vi "alligning data.vi"() -> (1 "Second part":waveform(dbl)[](graph), 2 "First Part":waveform(dbl)[](graph))   [LabVIEW 2020]
uses:
  <vilib>/measure/maresamp.llb/Resample Waveform (single shot).vi
  <vilib>/measure/maspectr.llb/FFT Spectrum (Real-Im) for 1 Chan.vi
  <vilib>/measure/NI_MAPro.lvlib
panel:
  out "Waveform Graph 6":cluster{"f0":dbl, "df":dbl, "real part":dbl[]}(graph)
  out "Delta second part 2":dbl
  out "Delta first part 2":dbl
  out "Delta second part":dbl
  out "Delta first part":dbl
  in  "Tab Control":enum32{"Page 1", "Page 3", "Page 4", "Page 2"}(tab)
  out "Waveform Graph 2":waveform(dbl)[](graph)
  out "Waveform Graph 3":waveform(dbl)[](graph)
  out "Array 4":i32[](array[numeric])
  out "Array 5":i32[](array[numeric])
  out "Waveform Graph 5":waveform(dbl)[](graph)
  out "Waveform Graph 4":waveform(dbl)[](graph)
  out "Array 2":i32[](array[numeric])
  out "Array 3":i32[](array[numeric])
  out "Array 7":i32[](array[numeric])
  out "Array 6":i32[](array[numeric])
  out "lv split cut":i32
  out "ex split cut":i32
  out "First ex cut":i32
  out "second subarray 2":dbl[](array[numeric])
  out "first subarray 2":dbl[](array[numeric])
  out "second subarray":dbl[](array[numeric])
  out "first subarray":dbl[](array[numeric])
  out "Array":i32[](array[numeric])
  out "x-y":dbl
  # "LV\nEX\nNew"
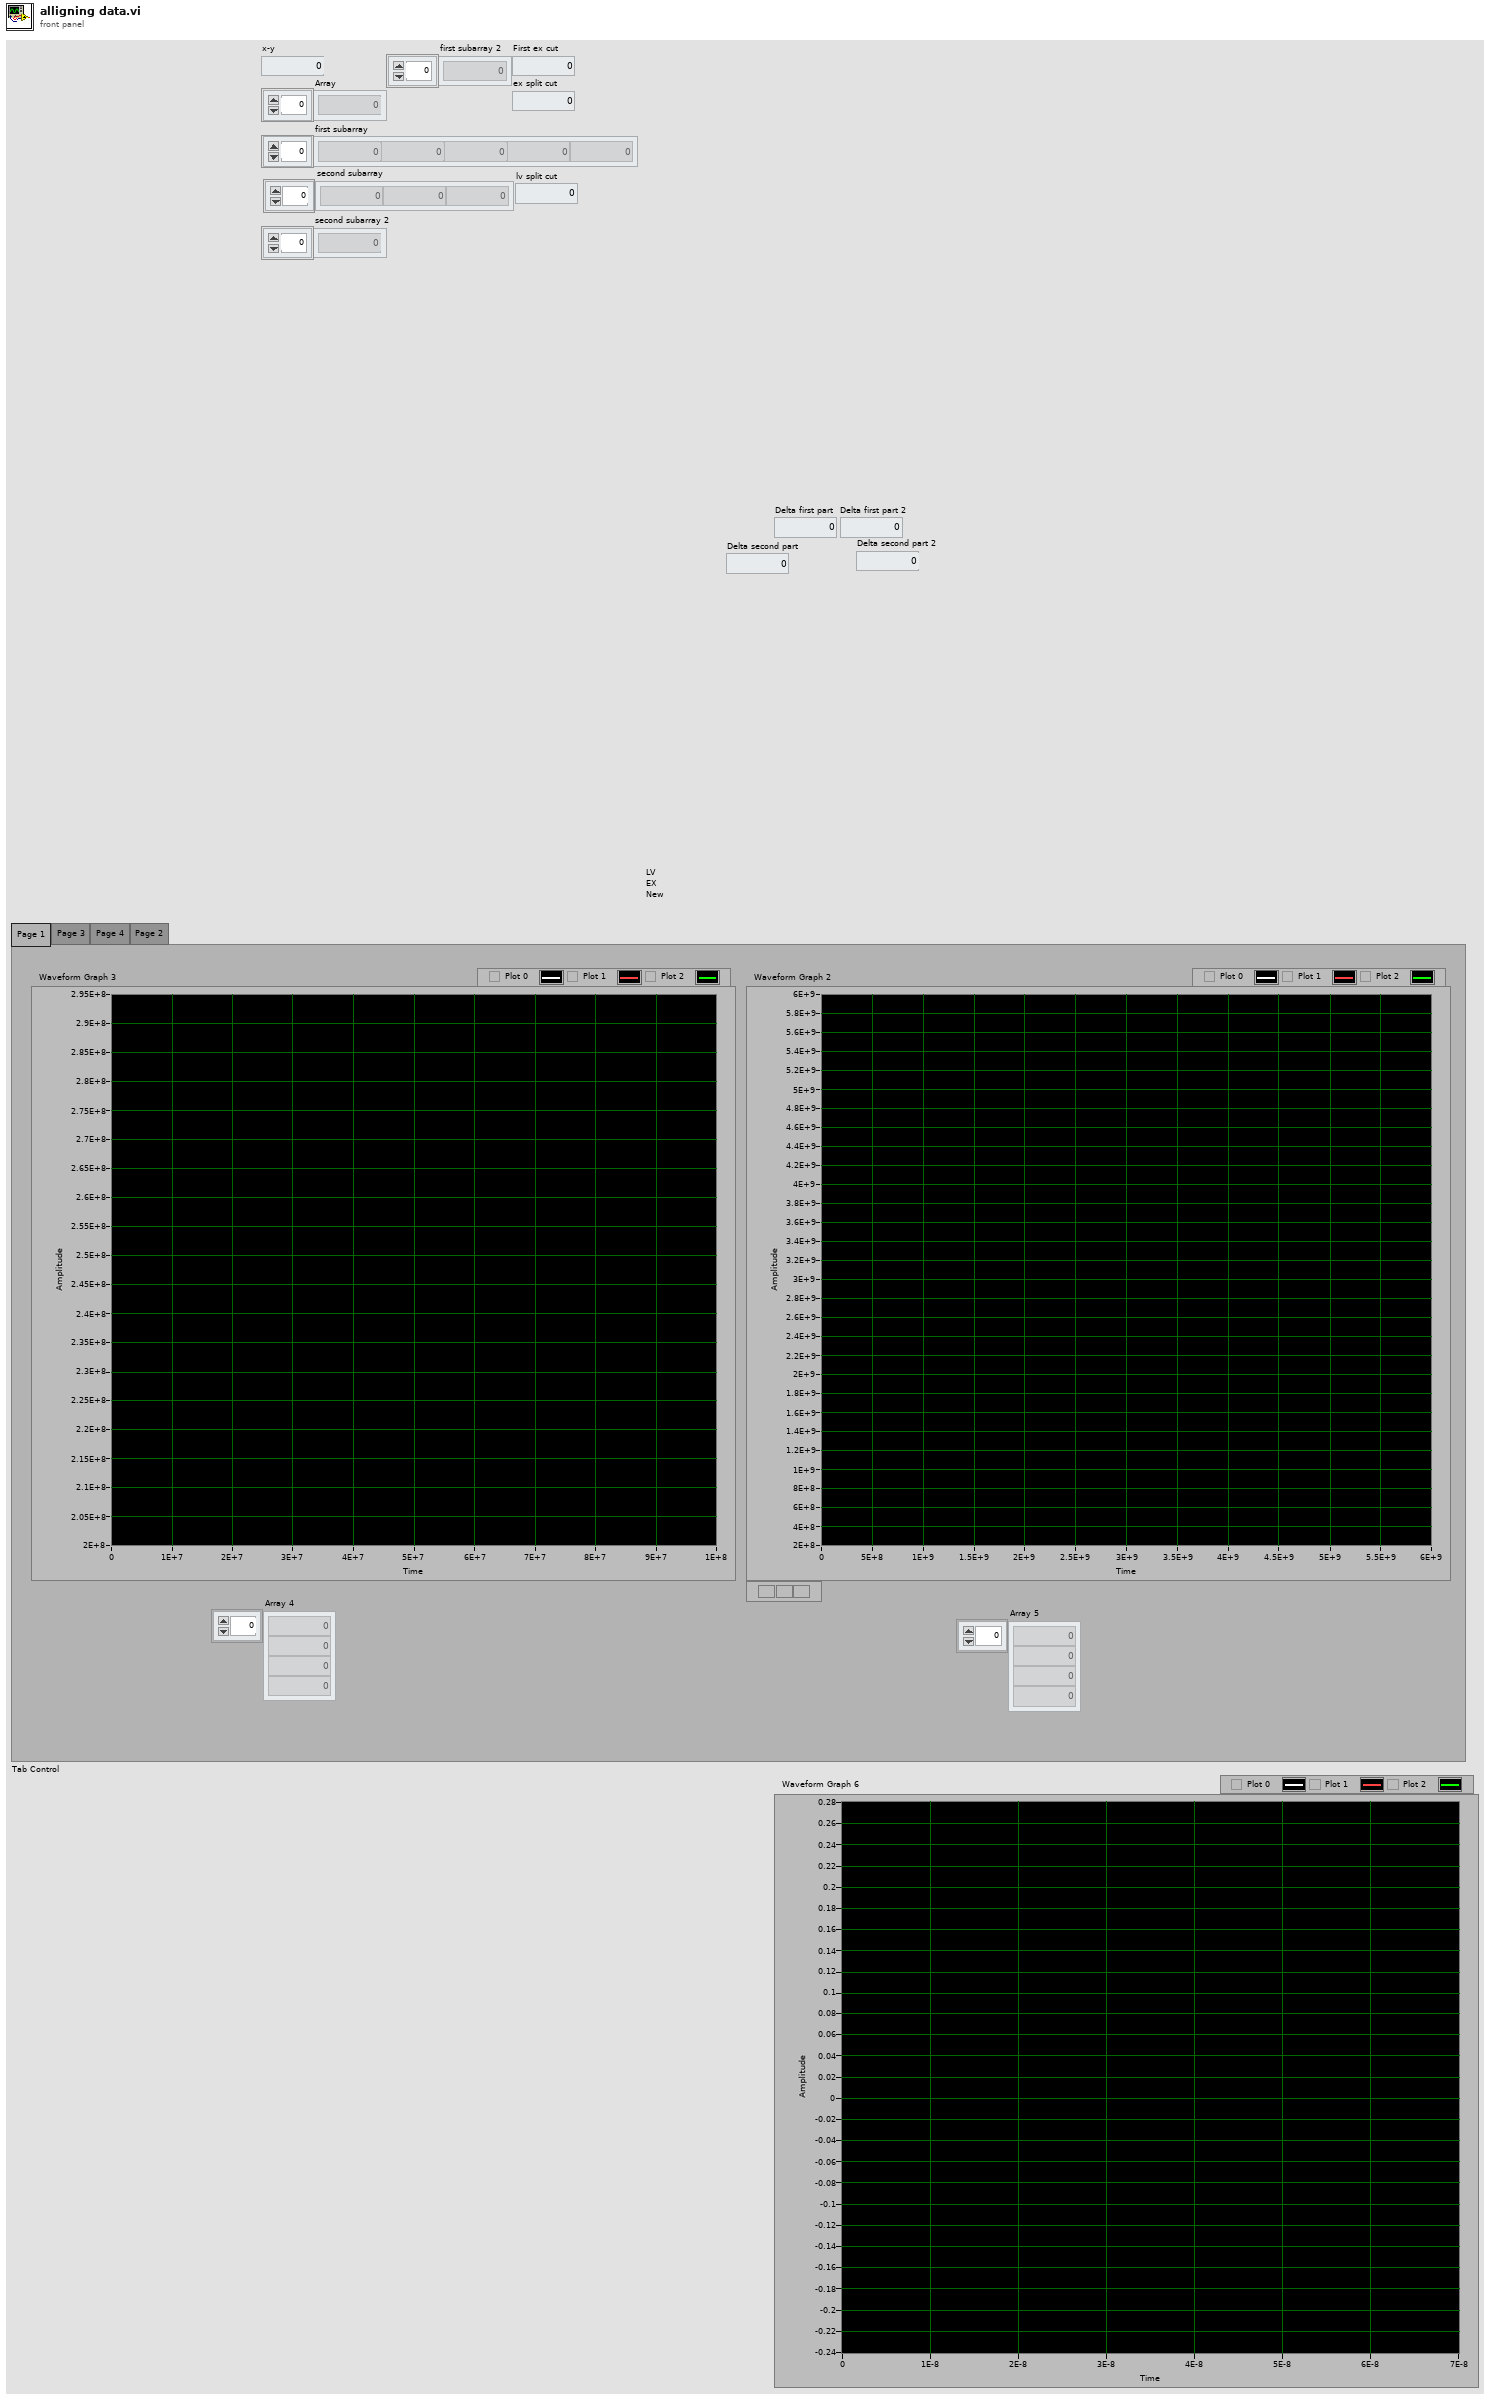
[diagram p1: front panel]
types:
  T1 = typedef "VFH-VNA_File_Handler.lvlib/VFH-file_cluster-Expensive.ctl" = cluster{"Frequency":dbl[], "Permativity'":dbl[], "Permativity''":dbl[], "Q [S/m]":dbl[], "Tan":dbl[], "Reflection R":dbl[], "Reflection I":dbl[]}
  T2 = typedef "VFH-VNA_File_Handler.lvlib/VFH-file_cluster-NanoVNA.ctl" = cluster{"Frequency":dbl[], "S11_Real":dbl[], "S11_Imag":dbl[], "S21_Real":dbl[], "S21_Imag":dbl[], "S12_Real":dbl[], "S12_Imag":dbl[], "S22_Real":dbl[], "S22_Imag":dbl[]}
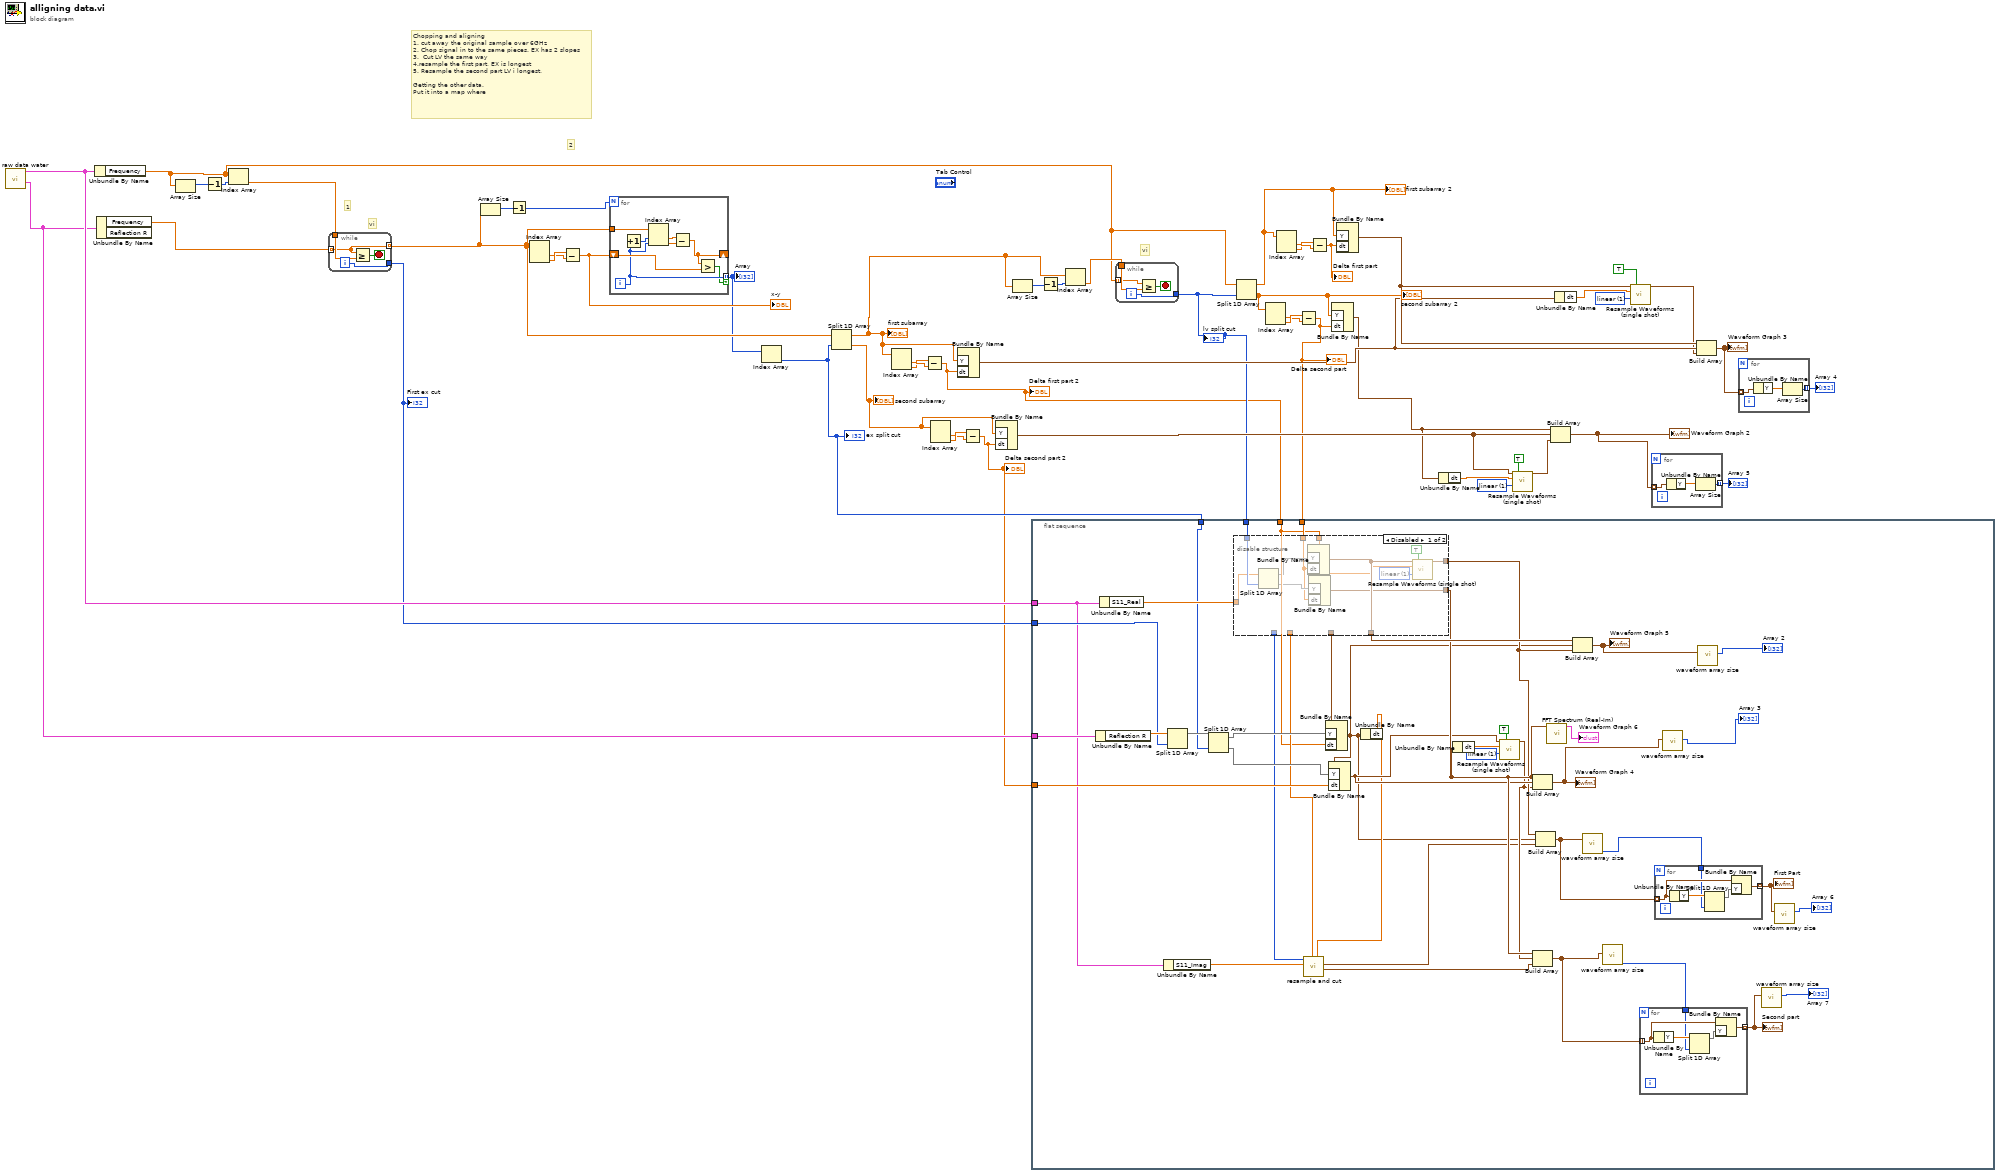
[diagram p0: block diagram]
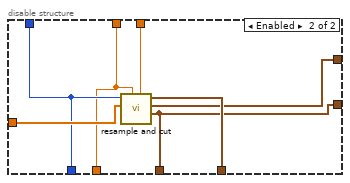
[diagram p2: hidden frame]
diagram:
  w17 = u16 1 items=["coerce", "linear", "spline", "FIR filter"] ("interpolation mode")
  w23 = u16 1 items=["coerce", "linear", "spline", "FIR filter"] ("interpolation mode")
  # "vi"
  # "vi"
  # "2"
  # "1"
  # "Chopping and aligning\n1. cut away the original sample over 6GHz \n2. Chop signal in to the same pieces. EX has 2 slopes\n3.  Cut LV the same way\n4.resample the first part, EX is longest\n5. Resample the second part LV i longest.\n\nGetting the other data.\nPut it into a map where"
  n1 = call "raw data water.vi"() -> ("output R140"=w11:T1, "avg output NV"=w12:T2)  [unwired: 9 in, 1 out]
  n2 = Unbundle By Name(w12) -> ("Frequency"=w38:dbl[])
  n3 = Unbundle By Name(w11) -> ("Frequency"=w49:dbl[])  [unwired: 1 out]
  n4 = Array Size(array=w38) -> (size(s)=w52:i32)
  n5 = Decrement(x=w52) -> (x-1=w51:i32)
  n6 = Index Array(array=w38, index=w51) -> (element=w50:dbl)
  n7 = while {
    tunnel: w49 -> [w54] mode=indexing
    tunnel: w50 -> [w56]
    tunnel: [w54] -> w43 mode=indexing
    tunnel: [w53] -> w10
    i -> [w53]
    stop <- w55 stop-if-true
    n8 = Greater Or Equal?(x=w54, y=w56) -> (x >= y?=w55:bool)
  }
  "First ex cut" <- w10
  n9 = Array Size(array=w43) -> (size(s)=w45:i32)
  n10 = Decrement(x=w45) -> (x-1=w44:i32)
  n11 = Index Array(array=w43) -> (element #1=w47:dbl, element #2=w48:dbl)  [unwired: 2 in]
  n12 = Subtract(x=w48, y=w47) -> (x-y=w46:dbl)
  "x-y" <- w46
  n13 = for {
    N: w44 -> [_]
    tunnel: w43 -> [w64]
    shift-right: [w60] -> _
    shift-left: w46 -> [w59]
    tunnel: [w58] -> w42 mode=indexing if=w57
    i -> [w58]
    n14 = Increment(x=w58) -> (x+1=w63:i32)
    n15 = Index Array(array=w64, index #1=w63, index #2=w58) -> (element #1=w62:dbl, element #2=w61:dbl)
    n16 = Subtract(x=w62, y=w61) -> (x-y=w60:dbl)
    n17 = Greater?(x=w60, y=w59) -> (0:w57:bool)
  }
  "Array" <- w42
  n18 = Index Array(array=w42) -> (element=w9:i32)  [unwired: 1 in]
  "ex split cut" <- w9
  n19 = Split 1D Array(array=w43, index=w9) -> (first subarray=w28:dbl[], second subarray=w25:dbl[])
  "first subarray" <- w28
  "second subarray" <- w25
  n20 = Index Array(array=w28) -> (element #1=w30:dbl, element #2=w29:dbl)  [unwired: 2 in]
  n21 = Subtract(x=w29, y=w30) -> (x-y=w6:dbl)
  "Delta first part 2" <- w6
  n22 = Index Array(array=w25) -> (element #1=w26:dbl, element #2=w27:dbl)  [unwired: 2 in]
  n23 = Bundle By Name("Y"=w28, "dt"=w6) -> (w21:waveform(dbl))  [unwired: 1 in]
  n24 = Subtract(x=w27, y=w26) -> (x-y=w5:dbl)
  "Delta second part 2" <- w5
  n25 = Bundle By Name("Y"=w25, "dt"=w5) -> (w15:waveform(dbl))  [unwired: 1 in]
  n26 = Array Size(array=w28) -> (size(s)=w40:i32)
  n27 = flat-sequence {
    tunnel: w12 -> [w75]
    tunnel: w11 -> [w106]
    tunnel: w10 -> [w94]
    tunnel: w9 -> [w93]
    tunnel: w8 -> [w98]
    tunnel: w7 -> [w103]
    tunnel: w6 -> [w68]
    tunnel: w5 -> [w102]
    frame #0 {
      w100 = u16 1 items=["coerce", "linear", "spline", "FIR filter"] ("interpolation mode")
      n28 = Unbundle By Name(w106) -> ("Reflection R"=w95:dbl[])
      n29 = Unbundle By Name(w75) -> ("S11_Real"=w97:dbl[])
      n30 = Unbundle By Name(w75) -> ("S11_Imag"=w74:dbl[])
      n31 = Split 1D Array(array=w95, index=w94) -> (first subarray=w96:dbl[])  [unwired: 1 out]
      n32 = Split 1D Array(array=w96, index=w93) -> (first subarray=w104:dbl[], second subarray=w105:dbl[])
      n33 = disable-structure shown="Disabled" {
        disable-tunnel: w103 -> [w113 w120]
        disable-tunnel: w98 -> [w112 w121]
        disable-tunnel: w97 -> [w111 w124]
        disable-tunnel: [w110 w123] -> w91
        disable-tunnel: [w109 w118] -> w90
        disable-tunnel: [w108 w122] -> w88
        disable-tunnel: [_ w121] -> w73
        disable-tunnel: [_ w120] -> w72
        disable-tunnel: w68 -> [w107 w119]
        disable-tunnel: [_ w118] -> w67
        frame Disabled {
          w114 = u16 1 items=["coerce", "linear", "spline", "FIR filter"] ("interpolation mode")
          n34 = Split 1D Array(array=w111, index=w112) -> (first subarray=w117:dbl[], second subarray=w116:dbl[])
          n35 = Bundle By Name("Y"=w117, "dt"=w113) -> (w110:waveform(dbl))  [unwired: 1 in]
          n36 = Bundle By Name("Y"=w116, "dt"=w113) -> (w109:waveform(dbl))  [unwired: 1 in]
          n37 = call-poly <vilib>:"Resample Waveforms (single shot).vi"("waveform in"=w110, "open interval? (F)"=TRUE, "dt"=w107, "interpolation mode"=w114) -> ("resampled waveform out"=w108:waveform(dbl))  [unwired: 8 in, 3 out]
        }
        frame Enabled {
          n38 = call "resample and cut.vi"("new dt"=w119, "signal dt"=w120, "array"=w124, "Splite"=w121) -> ("org second part"=w118:waveform(dbl), "resampled first part"=w122:waveform(dbl), "Org first part"=w123:waveform(dbl))  [unwired: 5 in]
        }
      }
      n39 = Bundle By Name(cluster=w67, "Y"=w104, "dt"=w68) -> (w66:waveform(dbl))
      n40 = Bundle By Name(cluster=w66, "Y"=w105, "dt"=w102) -> (w89:waveform(dbl))
      n41 = Unbundle By Name(w66) -> ("dt"=w71:dbl)
      n42 = call "resample and cut.vi"("new dt"=w71, "signal dt"=w72, "array"=w74, "Splite"=w73) -> ("org second part"=w69:waveform(dbl), "resampled first part"=w70:waveform(dbl))  [unwired: 5 in, 1 out]
      n43 = Unbundle By Name(w90) -> ("dt"=w101:dbl)
      n44 = call-poly <vilib>:"Resample Waveforms (single shot).vi"("waveform in"=w89, "open interval? (F)"=TRUE, "dt"=w101, "interpolation mode"=w100) -> ("resampled waveform out"=w87:waveform(dbl))  [unwired: 8 in, 3 out]
      n45 = Build Array(w90, w87, w69) -> (w81:waveform(dbl)[])
      n46 = Build Array(w90, w89, w87) -> (w84:waveform(dbl)[])
      "Waveform Graph 4" <- w84
      n47 = Build Array(w88, w66, w70) -> (w82:waveform(dbl)[])
      n48 = call-poly <vilib>:"FFT Spectrum (Real-Im).vi"("time signal"=w90) -> ("real part"=→"Waveform Graph 6":cluster{"f0":dbl, "df":dbl, "real part":dbl[]})  [unwired: 6 in, 4 out]
      n49 = Build Array(w91, w66, w88) -> (w86:waveform(dbl)[])
      "Waveform Graph 5" <- w86
      n50 = call "waveform array size.vi"("Waveform"=w82) -> ("min value"=w65:i32)  [unwired: 8 in, 2 out]
      n51 = call "waveform array size.vi"("Waveform"=w81) -> ("min value"=w80:i32)  [unwired: 8 in, 2 out]
      n52 = for {
        tunnel: w81 -> [w129] mode=indexing
        tunnel: w80 -> [w126]
        tunnel: [w125] -> w77 mode=indexing
        n53 = Unbundle By Name(w129) -> ("Y"=w128:dbl[])
        n54 = Split 1D Array(array=w128, index=w126) -> (first subarray=w127:dbl[])  [unwired: 1 out]
        n55 = Bundle By Name(cluster=w129, "Y"=w127) -> (w125:waveform(dbl))
      }
      "Second part" <- w77
      n56 = for {
        tunnel: w82 -> [w134] mode=indexing
        tunnel: w65 -> [w131]
        tunnel: [w130] -> w79 mode=indexing
        n57 = Unbundle By Name(w134) -> ("Y"=w133:dbl[])
        n58 = Split 1D Array(array=w133, index=w131) -> (first subarray=w132:dbl[])  [unwired: 1 out]
        n59 = Bundle By Name(cluster=w134, "Y"=w132) -> (w130:waveform(dbl))
      }
      "First Part" <- w79
      n60 = call "waveform array size.vi"("Waveform"=w84) -> ("Array"=→"Array 3":i32[])  [unwired: 8 in, 2 out]
      n61 = call "waveform array size.vi"("Waveform"=w86) -> ("Array"=→"Array 2":i32[])  [unwired: 8 in, 2 out]
      n62 = call "waveform array size.vi"("Waveform"=w77) -> ("Array"=→"Array 7":i32[])  [unwired: 8 in, 2 out]
      n63 = call "waveform array size.vi"("Waveform"=w79) -> ("Array"=→"Array 6":i32[])  [unwired: 8 in, 2 out]
    }
  }
  n64 = Decrement(x=w40) -> (x-1=w41:i32)
  n65 = Index Array(array=w28, index=w41) -> (element=w39:dbl)
  n66 = while {
    tunnel: w38 -> [w136] mode=indexing
    tunnel: w39 -> [w138]
    tunnel: [w135] -> w8
    i -> [w135]
    stop <- w137 stop-if-true
    n67 = Greater Or Equal?(x=w136, y=w138) -> (x >= y?=w137:bool)
  }
  "lv split cut" <- w8
  n68 = Split 1D Array(array=w38, index=w8) -> (first subarray=w33:dbl[], second subarray=w31:dbl[])
  "first subarray 2" <- w33
  "second subarray 2" <- w31
  n69 = Index Array(array=w31) -> (element #1=w34:dbl, element #2=w35:dbl)  [unwired: 2 in]
  n70 = Index Array(array=w33) -> (element #1=w37:dbl, element #2=w36:dbl)  [unwired: 2 in]
  n71 = Subtract(x=w35, y=w34) -> (x-y=w7:dbl)
  "Delta second part" <- w7
  n72 = Subtract(x=w36, y=w37) -> (x-y=w32:dbl)
  "Delta first part" <- w32
  n73 = Bundle By Name("Y"=w31, "dt"=w7) -> (w14:waveform(dbl))  [unwired: 1 in]
  n74 = Bundle By Name("Y"=w33, "dt"=w32) -> (w22:waveform(dbl))  [unwired: 1 in]
  n75 = Unbundle By Name(w14) -> ("dt"=w18:dbl)
  n76 = call-poly <vilib>:"Resample Waveforms (single shot).vi"("waveform in"=w15, "open interval? (F)"=TRUE, "dt"=w18, "interpolation mode"=w17) -> ("resampled waveform out"=w13:waveform(dbl))  [unwired: 8 in, 3 out]
  n77 = Build Array(w14, w15, w13) -> (w1:waveform(dbl)[])
  "Waveform Graph 2" <- w1
  n78 = Unbundle By Name(w21) -> ("dt"=w20:dbl)
  n79 = call-poly <vilib>:"Resample Waveforms (single shot).vi"("waveform in"=w22, "open interval? (F)"=TRUE, "dt"=w20, "interpolation mode"=w23) -> ("resampled waveform out"=w19:waveform(dbl))  [unwired: 8 in, 3 out]
  n80 = for {
    tunnel: w1 -> [w141] mode=indexing
    tunnel: [w139] -> w2 mode=indexing
    n81 = Unbundle By Name(w141) -> ("Y"=w140:dbl[])
    n82 = Array Size(array=w140) -> (size(s)=w139:i32)
  }
  "Array 5" <- w2
  n83 = Build Array(w22, w21, w19) -> (w3:waveform(dbl)[])
  "Waveform Graph 3" <- w3
  n84 = for {
    tunnel: w3 -> [w144] mode=indexing
    tunnel: [w142] -> w4 mode=indexing
    n85 = Unbundle By Name(w144) -> ("Y"=w143:dbl[])
    n86 = Array Size(array=w143) -> (size(s)=w142:i32)
  }
  "Array 4" <- w4
